vi "Check String is All ASCII.vi"(3 "string In":string) -> (1 "All is ASCII？":bool)   [LabVIEW 2021]
doc: "check the string is make up by ASCII.\n2016-05-19 14:49:05\n蒋松\nsina: @sushu1051"
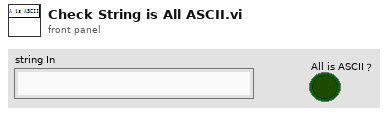
[diagram p1: front panel]
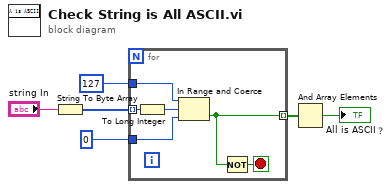
[diagram p0: block diagram]
diagram:
  n1 = String To Byte Array(string="string In") -> (unsigned byte array=w5:u8[])
  n2 = for {
    tunnel: w5 -> [w12] mode=indexing
    tunnel: 0 ("lower limit") -> [w9]
    tunnel: 127 ("upper limit") -> [w8]
    tunnel: [w7] -> w2 mode=indexing
    stop <- w10 stop-if-true
    n3 = To Long Integer(number=w12) -> (32bit integer=w11:i32)
    n4 = In Range and Coerce(upper limit=w8, x=w11, lower limit=w9) -> (In Range?=w7:bool)  [unwired: 1 out]
    n5 = Not(x=w7) -> (.not. x?=w10:bool)
  }
  n6 = And Array Elements(Boolean array=w2) -> (logical AND=→"All is ASCII？":bool)
